vi "add to repo.vi"(8 "error in":errorcluster, 9 "parent":string, 10 "serializable node":refnum<class "CEF_serializable node.lvclass">, 11 "CEF_HierarchyRepo in":refnum<class "CEF_HierarchyRepo.lvclass">) -> (0 "error out":errorcluster, 3 "CEF_HierarchyRepo out":refnum<class "CEF_HierarchyRepo.lvclass">)   [LabVIEW 2025, in "CEF.lvlib" / "CEF_HierarchyRepo.lvclass"]
doc: "Copyright 2017 National Instruments Corporation\n\nLicensed under the Apache License, Version 2.0 (the \"License\"); you may not use this file except in compliance with the License. You may obtain a copy of the License at http://www.apache.org/licenses/LICENSE-2.0\nUnless required by applicable law or agreed to in writing, software distributed under the License is distributed on an \"AS IS\" BASIS, WITHOUT WARRANTIES OR CONDITIONS OF ANY KIND, either express or implied. See the License for the specific language governing permissions and limitations under the License."
uses:
  CEF_HierarchyRepo.lvclass
  serializable node/CEF_serializable node.lvclass
  CEF_HierarchyRepo.lvclass/CEF_HierarchyRepo.ctl
  serializable configuration/CEF_serializable configuration.lvclass
  CEF.lvlib
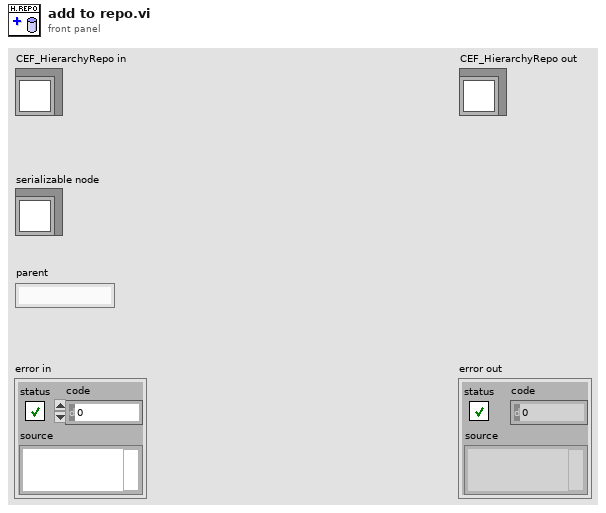
[diagram p1: front panel]
types:
  T1 = typedef "CEF.lvlib/CEF_HierarchyRepo.lvclass/memory hierarchy.ctl" = cluster{"hierarchy structure":T2, "instance data":refnum<class "CEF_serializable configuration.lvclass">[]}
  T2 = typedef "CEF.lvlib/CEF_HierarchyRepo.lvclass/full hierarchy.ctl" = cluster{"root":string, "hierarchy":T3[]}
  T3 = typedef "CEF.lvlib/hierarchy element.ctl" = cluster{"current node":string, "children":string[]}
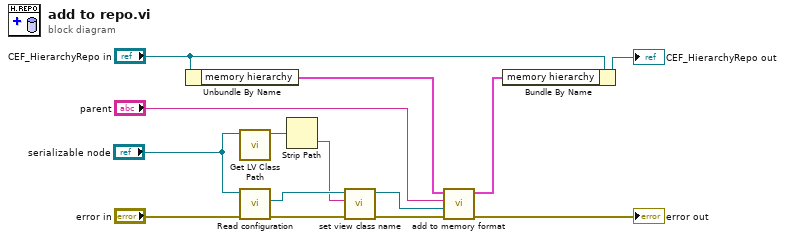
[diagram p0: block diagram]
diagram:
  n1 = Unbundle By Name("CEF_HierarchyRepo in") -> ("memory hierarchy"=w11:T1)
  n2 = call <vilib>:"Get LV Class Path.vi"("object"="serializable node") -> ("class path"=w7:path)  [unwired: 9 in, 1 out]
  n3 = call-dynamic "Read configuration.vi"("error in"="error in", "CEF_serializable node in"="serializable node") -> ("error out"=w1:errorcluster, "CEF Configuration"=w4:refnum<class "CEF_serializable configuration.lvclass">)  [unwired: 7 in, 1 out]
  n4 = Strip Path(path=w7) -> (name=w3:string)  [unwired: 1 out]
  n5 = call "set view class name.vi"("error in"=w1, "view class"=w3, "CEF_Configuration in"=w4) -> ("error out"=w6:errorcluster, "CEF_Configuration out"=w5:refnum<class "CEF_serializable configuration.lvclass">)  [unwired: 7 in]
  n6 = call "add to memory format.vi"("error in"=w6, "CEF_serializable configuration in"=w5, "parent ID"="parent", "memory hierarchy in"=w11) -> ("error out"=→"error out":errorcluster, "memory hierarchy out"=w13:T1)  [unwired: 6 in]
  n7 = Bundle By Name(cluster="CEF_HierarchyRepo in", "memory hierarchy"=w13) -> (→"CEF_HierarchyRepo out":refnum<class "CEF_HierarchyRepo.lvclass">)
